vi "ivory_os_send.vi"(8 "error in (no error)":errorcluster) -> (0 "error out":errorcluster)   [LabVIEW 2023]
panel:
  in  "anything":cluster{}
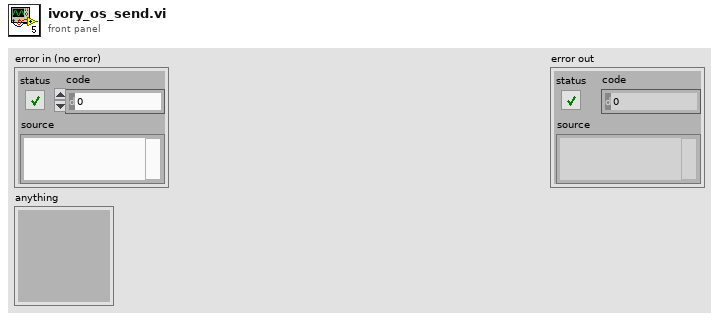
[diagram p1: front panel]
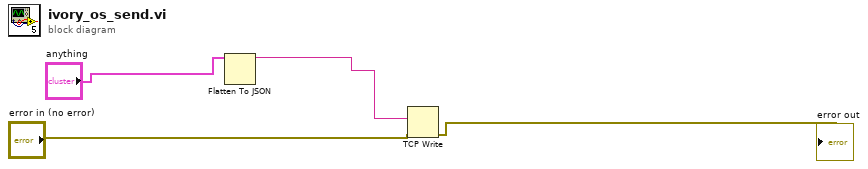
[diagram p0: block diagram]
diagram:
  n1 = Flatten To JSON(anything="anything") -> (JSON string=w3:string)  [unwired: 2 in, 1 out]
  n2 = TCP Write(data in=w3, error in (no error)="error in (no error)") -> (error out=→"error out":errorcluster)  [unwired: 2 in, 2 out]
